vi "check Abort.vi"(9 "timeout (0 ms)":i32, 11 "Job in":refnum<class "Job.lvclass">) -> (1 "exception":i32, 3 "Abort":bool)   [LabVIEW 2013, in "openCron.lvlib" / "Job.lvclass"]
uses:
  Job.lvclass
  Job.lvclass/Job.ctl
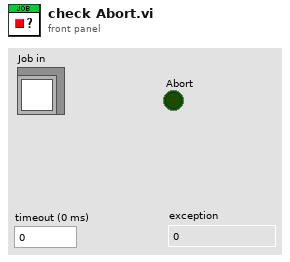
[diagram p1: front panel]
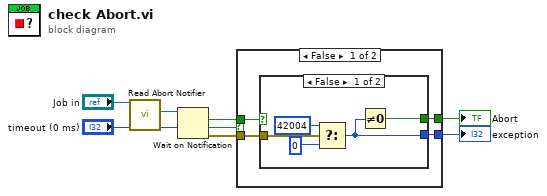
[diagram p0: block diagram]
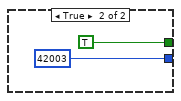
[diagram p2: hidden frame]
diagram:
  n1 = call "Read Abort Notifier.vi"("Job in"="Job in") -> ("Abort"=w3:refnum<notifier>)  [unwired: 10 in]
  n2 = Wait on Notification(notifier=w3, timeout in ms (-1)="timeout (0 ms)") -> (notification=w6:bool, timed out?=w1:bool, error out=w7:errorcluster)  [unwired: 2 in, 1 out]
  n3 = case shown="False" w1 {
    tunnel: [w12 _] -> w8
    tunnel: w7 -> [w11 _]
    tunnel: w6 -> [w10 _]
    tunnel: [w9 _] -> w5
    frame False {
      n4 = case shown="False" w10 {
        tunnel: [w13 42003 ("exception")] -> w9
        tunnel: w11 -> [w17 _]
        tunnel: [w14 TRUE] -> w12
        frame False {
          n5 = Select(t=42004, s=w17, f=0 ("exception")) -> (s? t:f=w13:i32)
          n6 = Not Equal To 0?(x=w13) -> (x != 0?=w14:bool)
        }
        frame True {
        }
      }
    }
    frame True {
    }
  }
  "Abort" <- w8
  "exception" <- w5
